vi "ForceFieldSpringyWallsDebounced.vi"(0 "Control point on body":dbl[](array[numeric]), 1 "Center":dbl[](array[numeric]), 2 "Bounds X":dbl[](array[numeric]), 3 "Force field active last cycle":bool, 4 "ForceZ and Moments":dbl[](array[numeric]), 6 "ForceFieldConstK":dbl, 10 "BoundsY":dbl[](array[numeric])) -> (7 "DesiredFM_FF":dbl[](array[numeric]), 9 "ActiveFF":bool)   [LabVIEW 2017]
uses:
  <vilib>/imath/engines/lvmath2/RunTimeEngine/Managers/WorkSpace/UID Generator.vi
  <vilib>/imath/engines/lvmath2/RunTimeEngine/BuiltInFunctions/is_inpolygon/NIMS_is_inpolygon(V).vi
  <vilib>/imath/engines/lvmath2/RunTimeEngine/RunTimeType/NIMS_RunTimeType_From StrictType (excl LVString).vi
  <instcachedir>/0/NIMS_RunTimeType_From StrictType (excl LVString)_1019F277F0A747EDBCA0F6C52CA54500.lvgen/NIMS_RunTimeType_From StrictType (excl LVString)_1019F277F0A747EDBCA0F6C52CA54500_000.vi
  <vilib>/imath/engines/lvmath2/RunTimeEngine/RunTimeType/NIMS_RunTimeType_Set Source Original Bool.vi
  <vilib>/imath/engines/lvmath2/RunTimeEngine/ErrorHandling/NIMS_Error From Error Code.vi
  <vilib>/imath/engines/lvmath2/RunTimeEngine/LocalVariableDefStatement/MC_LocalVariableDefStatement_Display.vi
  <vilib>/imath/engines/lvmath2/RunTimeEngine/Managers/SymbolTable/Clear UID.vi
  <vilib>/imath/engines/lvmath2/RunTimeEngine/NodeEndStatement/NIMS_NodeEndStatement_Output.vi
  <instcachedir>/0/NIMS_NodeEndStatement_Output_53EC0D466D134D7ABD903AC30B43404B.lvgen/NIMS_NodeEndStatement_Output_53EC0D466D134D7ABD903AC30B43404B_013.vi
  <vilib>/imath/engines/lvmath2/RunTimeEngine/ErrorHandling/NIMS_Finalize Error.vi
  <vilib>/imath/engines/lvmath2/RunTimeEngine/Managers/SymbolTable/NIMS_WorkSpace.lvlib
panel:
  in  "Debounce boundary scale constant":dbl
  out "Current_point":dbl[](array[numeric])
  out "center position":dbl[](array[numeric])
  # "Irregular Force Field"
  # "INPUTS"
  # "Irregular FF Boundary Pts"
  # "OUTPUTS:"
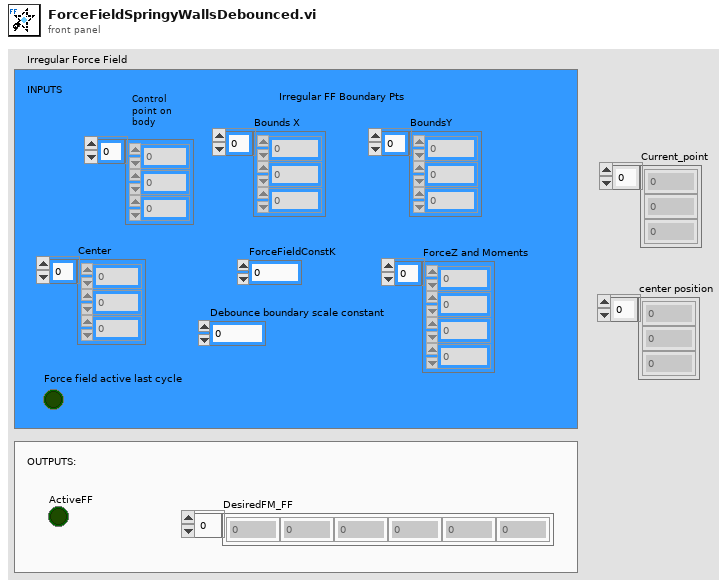
[diagram p1: front panel]
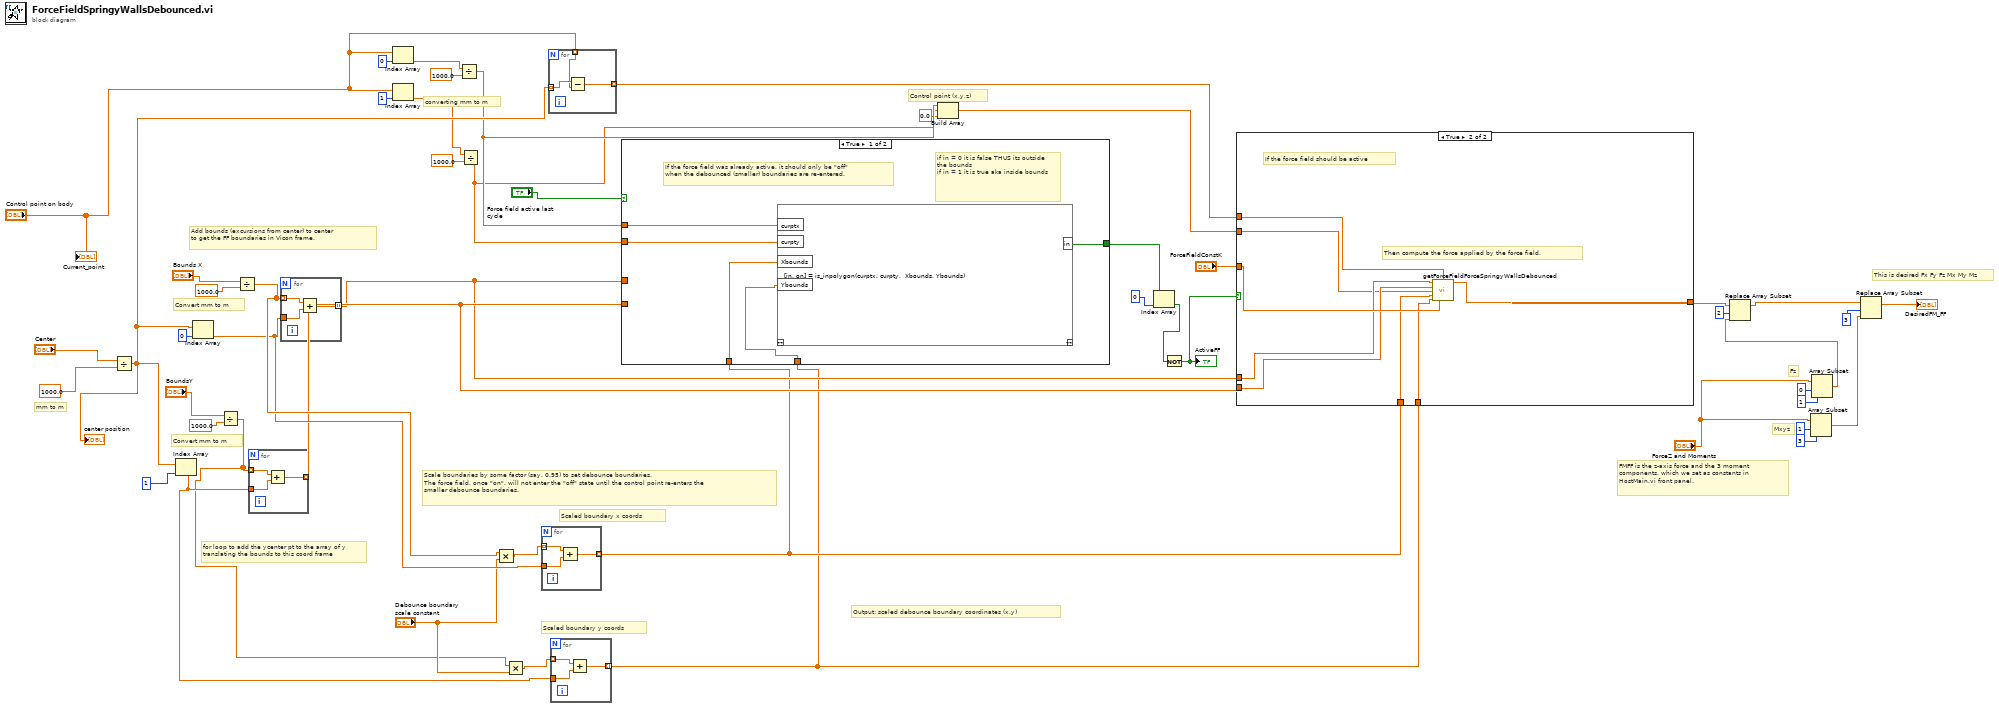
[diagram p0: block diagram]
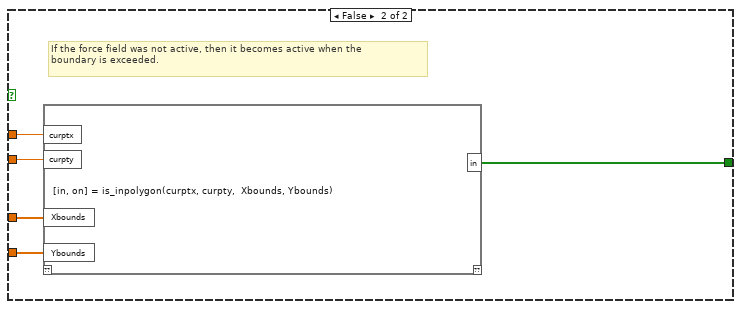
[diagram p2: hidden frame]
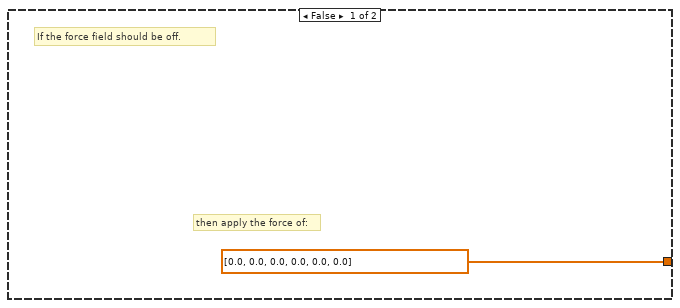
[diagram p3: hidden frame]
diagram:
  # "Control point (x,y,z)"
  # "FMFF is the z-axis force and the 3 moment \ncomponents, which we set as constants in \nHostMain.vi front panel."
  # "Add bounds (excursions from center) to center\nto get the FF boundaries in Vicon frame."
  # "Scaled boundary y coords"
  # "Scaled boundary x coords"
  # "Output: scaled debounce boundary coordinates (x,y)"
  # "Scale boundaries by some factor (say, 0.95) to set debounce boundaries.\nThe force field, once \"on\", will not enter the \"off\" state until the control point re-enters the\nsmaller debounce boundaries."
  # "Convert mm to m"
  # "Convert mm to m"
  # "for loop to add the ycenter pt to the array of y\ntranslating the bounds to this coord frame"
  # "This is desired Fx Fy Fz Mx My Mz"
  # "converting mm to m"
  # "Fz"
  # "Mxyz"
  # "mm to m"
  n1 = Divide(x="Center", y=1000.0) -> (x/y=w32:dbl[])
  "center position" <- w32
  n2 = Index Array(array=w32, index=1) -> (element=w20:dbl)
  n3 = Index Array(array=w32, index=0) -> (element=w22:dbl)
  n4 = Divide(x="BoundsY", y=1000.0) -> (x/y=w18:dbl[])
  n5 = Divide(x="Bounds X", y=1000.0) -> (x/y=w24:dbl[])
  n6 = for {
    tunnel: w20 -> [w53]
    tunnel: w18 -> [w52] mode=indexing
    tunnel: [w51] -> w17 mode=indexing
    n7 = Add(x=w52, y=w53) -> (x+y=w51:dbl)
  }
  n8 = for {
    tunnel: w22 -> [w56]
    tunnel: w24 -> [w55] mode=indexing
    tunnel: [w54] -> w16 mode=indexing
    n9 = Add(x=w55, y=w56) -> (x+y=w54:dbl)
  }
  n10 = Index Array(array="Control point on body", index=0) -> (element=w7:dbl)
  n11 = Index Array(array="Control point on body", index=1) -> (element=w5:dbl)
  n12 = Divide(x=w7, y=1000.0) -> (x/y=w4:dbl)
  n13 = Divide(x=w5, y=1000.0) -> (x/y=w3:dbl)
  n14 = Multiply(x=w24, y="Debounce boundary scale constant") -> (x*y=w23:dbl[])
  n15 = Multiply(x=w18, y="Debounce boundary scale constant") -> (x*y=w21:dbl[])
  n16 = for {
    tunnel: w22 -> [w59]
    tunnel: w23 -> [w58] mode=indexing
    tunnel: [w57] -> w11 mode=indexing
    n17 = Add(x=w58, y=w59) -> (x+y=w57:dbl)
  }
  n18 = for {
    tunnel: w32 -> [w61] mode=indexing
    tunnel: "Control point on body" -> [w60] mode=indexing
    tunnel: [w62] -> w31 mode=indexing
    n19 = Subtract(x=w61, y=w60) -> (x-y=w62:dbl)
  }
  n20 = for {
    tunnel: w20 -> [w65]
    tunnel: w21 -> [w64] mode=indexing
    tunnel: [w63] -> w10 mode=indexing
    n21 = Add(x=w64, y=w65) -> (x+y=w63:dbl)
  }
  n22 = case shown="True" "Force field active last cycle" {
    tunnel: [w70 w144] -> w14
    tunnel: w4 -> [w69 w143]
    tunnel: w3 -> [w68 w142]
    tunnel: w17 -> [_ w141]
    tunnel: w16 -> [_ w140]
    tunnel: w11 -> [w67 _]
    tunnel: w10 -> [w66 _]
    frame True {
      # "if in = 0 it is false THUS its outside the bounds\nif in = 1 it is true aka inside bounds"
      # "If the force field was already active, it should only be \"off\"\nwhen the debounced (smaller) boundaries are re-entered."
      n23 = mathscript code="[in, on] = is_inpolygon(curptx, curpty,  Xbounds, Ybounds)"("Xbounds"=w67, "Ybounds"=w66, "curptx"=w69, "curpty"=w68) -> ("in"=w70:bool[])  [unwired: 1 in, 1 out]
    }
    frame False {
      # "If the force field was not active, then it becomes active when the \nboundary is exceeded."
      n24 = mathscript code="[in, on] = is_inpolygon(curptx, curpty,  Xbounds, Ybounds)"("Xbounds"=w140, "Ybounds"=w141, "curptx"=w143, "curpty"=w142) -> ("in"=w144:bool[])  [unwired: 1 in, 1 out]
    }
  }
  n25 = Build Array(w4, w3, 0.0 ("element")) -> (w1:dbl[])
  n26 = Index Array(array=w14, index=0) -> (element=w13:bool)
  n27 = Not(x=w13) -> (.not. x?=w9:bool)
  "ActiveFF" <- w9
  n28 = case shown="True" w9 {
    tunnel: [dbl[] [0.0, 0.0, 0.0, 0.0, 0.0, 0.0] w220] -> w39
    tunnel: w31 -> [_ w221]
    tunnel: "ForceFieldConstK" -> [_ w222]
    tunnel: w17 -> [_ w219]
    tunnel: w16 -> [_ w218]
    tunnel: w11 -> [_ w217]
    tunnel: w10 -> [_ w216]
    tunnel: w1 -> [_ w215]
    frame False {
      # "then apply the force of:"
      # "If the force field should be off."
    }
    frame True {
      # "Then compute the force applied by the force field."
      # "If the force field should be active"
      n29 = call "getForceFieldForceSpringyWallsDebounced.vi"("Boundary X coords"=w218, "Desired force direction vector"=w221, "Boundary Y coords"=w219, "Current control point coordinates"=w215, "Scaled debounce boundary X coords"=w217, "Scaled debounce boundary Y coords"=w216, "forceScalingConstantK"=w222) -> ("Output FX FY Fz 0 0 0"=w220:dbl[])  [unwired: 8 in]
    }
  }
  n30 = Array Subset(array="ForceZ and Moments", index=1, length=3) -> (w41:dbl[])
  n31 = Array Subset(array="ForceZ and Moments", index=0, length=1) -> (w40:dbl[])
  n32 = Replace Array Subset(array=w39, new element=w40, index=2) -> (w47:dbl[])
  n33 = Replace Array Subset(array=w47, new element=w41, index=3) -> (→"DesiredFM_FF":dbl[])
  "Current_point" <- "Control point on body"
